vi "Pane Relief QD.vi"(6 "Variant in":variant, 7 "Shift Pressed?":bool, 8 "error in (no error)":errorcluster, 10 "QD Combo Box Ref":refnum<vi>, 11 "QD Launch VI Ref":refnum<vi>) -> (0 "error out":errorcluster, 4 "Variant out":variant)   [LabVIEW 2017]
doc: "Launches Pane Relief UI\n\nDefault Shortcut - [a]"
uses:
  Typedefs/Selection Colors--Cluster.ctl
  Classes/Pane Relief Main UI/Pane Relief Main UI/Pane Relief Main UI.lvclass
  C:/Program Files (x86)/National Instruments/LabVIEW 2017/vi.lib/MNProjects/Panel Manager/panel-actors/Source/Panel Actor/Panel Actor.lvclass
  <vilib>/MNProjects/Panel Manager/panel-actors/Source/Launch Root Panel Window.vi
  <vilib>/MNProjects/Panel Manager/panel-manager/Source/Window Position/Persistent Position/Persistent Position.vi
  <vilib>/MNProjects/Panel Manager/panel-manager/Source/MGI-Panel Manager.lvlib
  <vilib>/MNProjects/Panel Manager/panel-manager/Source/Window Position/Persistent Position/Persistent Position.lvclass
  <vilib>/MNProjects/Panel Manager/panel-actors/Source/MGI-Panel Actor.lvlib
  C:/Program Files (x86)/National Instruments/LabVIEW 2017/vi.lib/ActorFramework/Actor/Actor.lvclass
panel:
  in  "Undo Name":string="Quick Drop Keyboard Shortcut"
  # "Do not change the connector pane of this VI.\n\nSee the block diagram for directions on how to use this template."
  # "Specify the name of the Undo transaction"
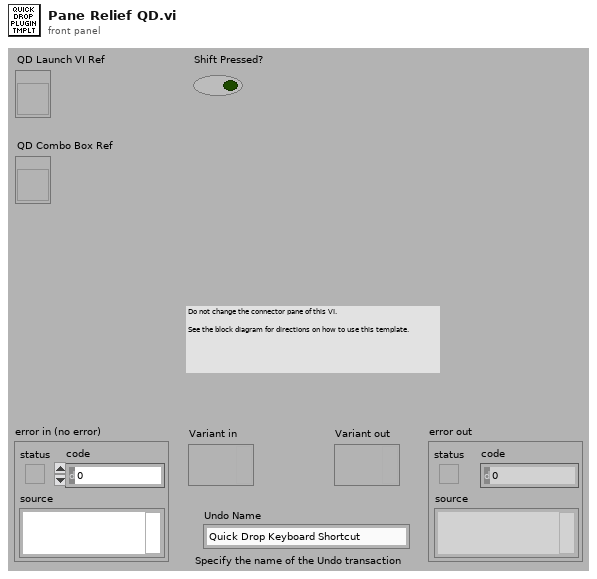
[diagram p1: front panel]
types:
  T1 = typedef "Selection Colors--Cluster.ctl" = cluster{"Normal":u32, "Mouse-over":u32, "Selected":u32, "Selected Mouse-over":u32}
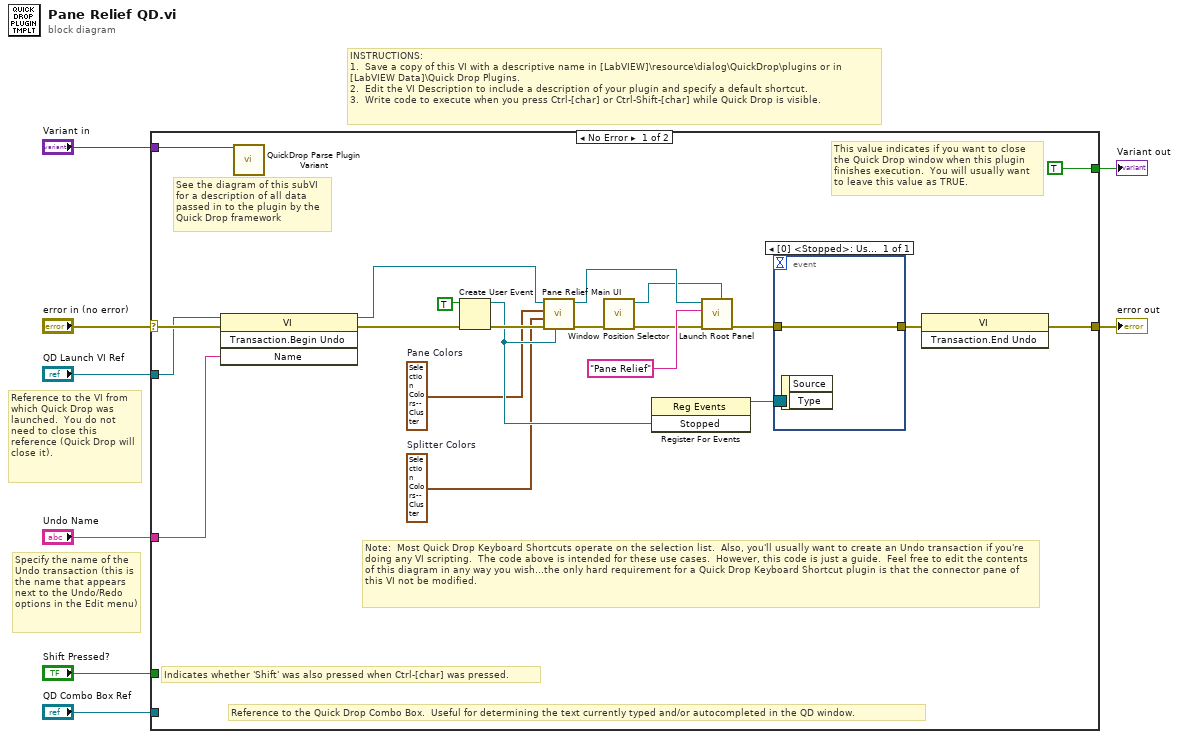
[diagram p0: block diagram]
diagram:
  # "Specify the name of the Undo transaction (this is the name that appears next to the Undo/Redo options in the Edit menu)"
  # "Reference to the VI from which Quick Drop was launched.  You do not need to close this reference (Quick Drop will close it)."
  # "INSTRUCTIONS:\n1.  Save a copy of this VI with a descriptive name in [LabVIEW]\\resource\\dialog\\QuickDrop\\plugins or in [LabVIEW Data]\\Quick Drop Plugins.\n2.  Edit the VI Description to include a description of your plugin and specify a default shortcut. \n3.  Write code to execute when you press Ctrl-[char] or Ctrl-Shift-[char] while Quick Drop is visible."
  n1 = case shown="No Error" "error in (no error)" {
    selector: "error in (no error)" -> [w27 w31]
    tunnel: [w26 w31] -> w7
    tunnel: "QD Launch VI Ref" -> [w25 _]
    tunnel: "Shift Pressed?" -> [_ _]
    tunnel: "QD Combo Box Ref" -> [_ _]
    tunnel: "Variant in" -> [w29 _]
    tunnel: "Undo Name" -> [w24 _]
    tunnel: [TRUE _] -> w1
    frame No Error {
      w10 = T1 {"Normal"=13620442, "Mouse-over"=12304582, "Selected"=3245000, "Selected Mouse-over"=1011636}  # Pane Colors
      w9 = T1 {"Normal"=8818326, "Mouse-over"=7502466, "Selected"=1994152, "Selected Mouse-over"=741250}  # Splitter Colors
      # "Note:  Most Quick Drop Keyboard Shortcuts operate on the selection list.  Also, you'll usually want to create an Undo transaction if you're doing any VI scripting.  The code above is intended for these use cases.  However, this code is just a guide.  Feel free to edit the contents of this diagram in any way you wish...the only hard requirement for a Quick Drop Keyboard Shortcut plugin is that the connector pane of this VI not be modified."
      # "This value indicates if you want to close the Quick Drop window when this plugin finishes execution.  You will usually want to leave this value as TRUE."
      # "See the diagram of this subVI for a description of all data passed in to the plugin by the Quick Drop framework"
      # "Reference to the Quick Drop Combo Box.  Useful for determining the text currently typed and/or autocompleted in the QD window."
      # "Indicates whether 'Shift' was also pressed when Ctrl-[char] was pressed."
      n2 = invoke class="VI" method="Transaction.Begin Undo"(reference=w25, error in=w27, "Name"=w24) -> (reference out=w12:refnum<vi>, error out=w13:errorcluster)  [unwired: 1 in, 2 out]
      n3 = call <vilib>:"QuickDrop Parse Plugin Variant.vi"("QDKS Variant in"=w29) -> ()  [unwired: 12 in, 3 out]
      n4 = Create User Event(user event datatype=TRUE ("Stopped"), error in=w13) -> (user event=w11:refnum<user-event>, error out=w17:errorcluster)
      n5 = call "Pane Relief Main UI.vi"("Stopped Event"=w11, "Error In"=w17, "Splitter Colors"=w9, "Pane Colors"=w10, "QD Launch VI Ref"=w12) -> ("Error Out"=w20:errorcluster, "Pane Relief Main UI out"=w23:refnum<class "Pane Relief Main UI.lvclass">)  [unwired: 5 in]
      n6 = call-poly <vilib>:"Window Position Selector.vi"("Error In"=w20) -> ("Error Out"=w19:errorcluster, "Persistent Position out"=w22:refnum<class "Window Position.lvclass">)  [unwired: 9 in]
      n7 = register-events(w11) -> (reference out=w14:refnum<event-registration>)  [unwired: 2 in, 1 out]
      n8 = call-poly <vilib>:"Launch Root Panel.vi"("Window Position (Maximize First Call)"=w22, "Error In"=w19, "Title"="Pane Relief", "Panel Actor in"=w23) -> ("Error Out"=w15:errorcluster)  [unwired: 6 in, 1 out]
      n9 = event shown="[0] <Stopped>: User Event" {
        selector: w14 -> [_]
        dyn-events: _ -> [_]
        timeout: _ -> [_]
        tunnel: [w30] -> w16
        tunnel: w15 -> [w30]
        event User Event {
          n10 = event-data() -> ()  [unwired: 1 in, 2 out]
        }
      }
      n11 = invoke class="VI" method="Transaction.End Undo"(error in=w16) -> (error out=w26:errorcluster)  [unwired: 2 in, 2 out]
    }
    frame Error {
    }
  }
  "error out" <- w7
  "Variant out" <- w1
